vi "DAC_convert_time-to-FPGA-timing.vi"(11 "time (ms)":sgl) -> (2 "p":fxp<+,11,11>, 3 "n":fxp<+,5,5>)   [LabVIEW 2013]
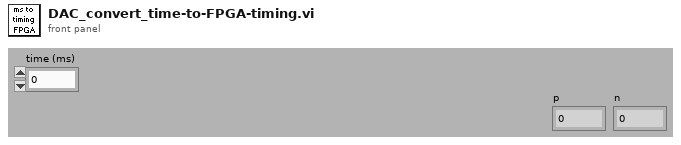
[diagram p1: front panel]
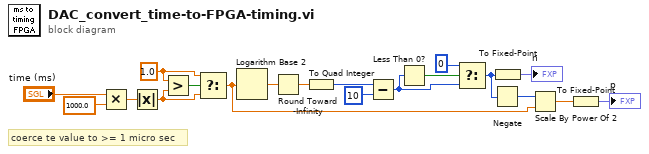
[diagram p0: block diagram]
diagram:
  w5 = sgl 1.0 ("t")
  # "coerce te value to >= 1 micro sec"
  n1 = Multiply(x="time (ms)", y=sgl 1000.0) -> (x*y=w13:sgl)
  n2 = Absolute Value(x=w13) -> (abs(x)=w7:sgl)
  n3 = Greater?(x=w5, y=w7) -> (0:w8:bool)
  n4 = Select(t=w5, s=w8, f=w7) -> (s? t:f=w6:sgl)
  n5 = Logarithm Base 2(1:w6) -> (0:w19:sgl)
  n6 = Round Toward -Infinity(1:w19) -> (0:w18:sgl)
  n7 = To Quad Integer(1:w18) -> (0:w17:i64)
  n8 = Subtract(x=w17, y=i64 10) -> (x-y=w10:i64)
  n9 = Less Than 0?(x=w10) -> (x < 0?=w11:bool)
  n10 = Select(t=i64 0, s=w11, f=w10) -> (s? t:f=w4:i64)
  n11 = Negate(x=w4) -> (-x=w14:i64)
  n12 = To Fixed-Point(number=w4) -> (fixed-point=→"n":fxp<+,5,5>)  [unwired: 1 out]
  n13 = Scale By Power Of 2(n=w14, x=w6) -> (x*2^n=w3:sgl)
  n14 = To Fixed-Point(number=w3) -> (fixed-point=→"p":fxp<+,11,11>)  [unwired: 1 out]
